vi "ActivateMenu.vi"(7 "Menu.lvclass":refnum<class "Menu.lvclass">, 8 "error in (no error)":errorcluster caption="错误输入（无错误）", 9 "MenuClassArray":refnum<class "Menu.lvclass">[](array[class]), 11 "listbox 输入":refnum<class "listbox.lvclass">) -> (0 "error out":errorcluster caption="错误输出", 3 "listbox 输出":refnum<class "listbox.lvclass">)   [LabVIEW 2016, in "listbox.lvclass"]
uses:
  listbox.lvclass
  LNK/Parent Class/Menu.lvclass
  listbox.lvclass/listbox.ctl
  LNK/Parent Class/Menu.lvclass/Menu.ctl
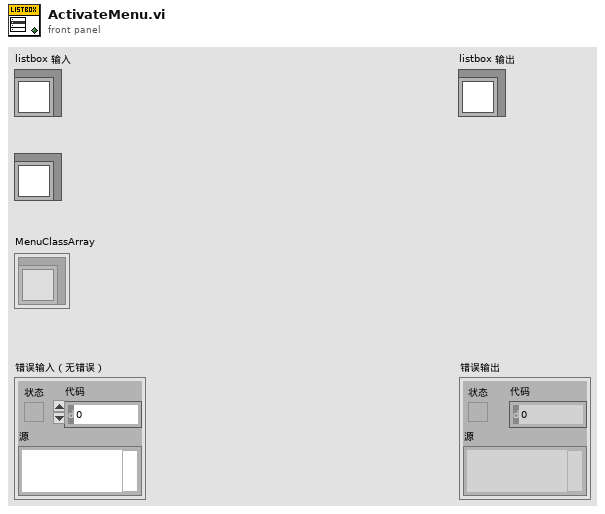
[diagram p1: front panel]
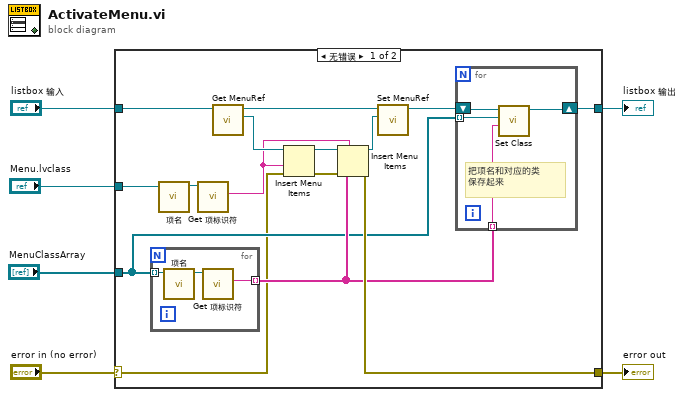
[diagram p0: block diagram]
diagram:
  n1 = case shown="无错误" "error in (no error)" {
    selector: "error in (no error)" -> [w8 w30]
    tunnel: [w16 w30] -> w5
    tunnel: [w14 w29] -> w3
    tunnel: "listbox 输入" -> [w21 w29]
    tunnel: "Menu.lvclass" -> [w18 _]
    tunnel: "MenuClassArray" -> [w12 _]
    frame No Error {
      n2 = for {
        tunnel: w12 -> [w28] mode=indexing
        tunnel: [w26] -> w13 mode=indexing
        n3 = call-dynamic "项名.vi"("LNK 输入"=w28) -> ("LNK 输出"=w27:refnum<class "Menu.lvclass">)  [unwired: 9 in, 1 out]
        n4 = call "Get 项标识符.vi"("LNK in"=w27) -> ("项标识符"=w26:string)  [unwired: 9 in, 1 out]
      }
      n5 = call-dynamic "项名.vi"("LNK 输入"=w18) -> ("LNK 输出"=w19:refnum<class "Menu.lvclass">)  [unwired: 9 in, 1 out]
      n6 = call "Get 项标识符.vi"("LNK in"=w19) -> ("项标识符"=w9:string)  [unwired: 9 in, 1 out]
      n7 = call "Get MenuRef.vi"("listbox in"=w21) -> ("MenuRef"=w11:refnum<k9>, "listbox out"=w20:refnum<class "listbox.lvclass">)  [unwired: 9 in]
      n8 = Insert Menu Items(6:w8, 7:w9, 9:w11) -> (0:w7:errorcluster, 3:w10:refnum<k9>)  [unwired: 3 in, 1 out]
      n9 = Insert Menu Items(5:w9, 6:w7, 7:w13, 9:w10) -> (0:w16:errorcluster, 3:w17:refnum<k9>)  [unwired: 2 in, 1 out]
      n10 = call "Set MenuRef.vi"("MenuRef"=w17, "listbox in"=w20) -> ("listbox out"=w15:refnum<class "listbox.lvclass">)  [unwired: 9 in]
      n11 = for {
        shift-right: [w24] -> w14
        shift-left: w15 -> [w25]
        tunnel: w13 -> [w23] mode=indexing
        tunnel: w12 -> [w22] mode=indexing
        # "把项名和对应的类\n保存起来"
        n12 = call "Set Class.vi"("项标识符"=w23, "LNK.lvclass"=w22, "listbox 输入"=w25) -> ("listbox 输出"=w24:refnum<class "listbox.lvclass">)  [unwired: 7 in, 1 out]
      }
    }
    frame Error {
    }
  }
  "error out" <- w5
  "listbox 输出" <- w3
